vi "GPI_MODE - Type.vi"(8 "error in (no error)":errorcluster, 11 "GPI_MODE":T1) -> (0 "error out":errorcluster, 3 "GPI_MODE_VALUE":i32)   [LabVIEW 2013]
doc: "<b>GPI port state options</b>\nOFF : Input off.\nTRIGGER : Trigger input.\nEXT_EVENT : External signal input."
uses:
  GPI_MODE.ctl
  C:/Projects/Cameras3.x/xiLib/xiLIB_64bit/xiLIB/xiCamLib/API/x64/xiApi.NETX64.dll
  xiLIB_64bit/xiLIB/xiCamLib/API/x64/xiApi.NETX64.dll
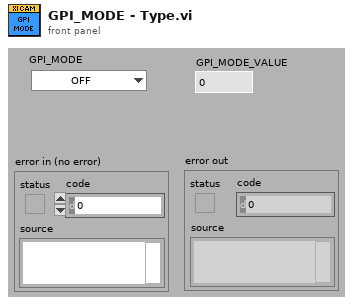
[diagram p1: front panel]
types:
  T1 = typedef "GPI_MODE.ctl" = enum16{"OFF", "TRIGGER", "EXT_EVENT"}
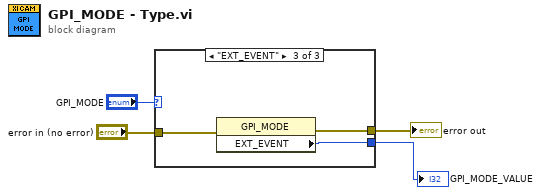
[diagram p0: block diagram]
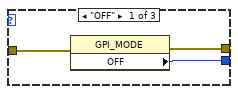
[diagram p2: hidden frame]
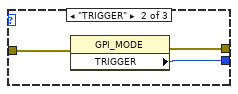
[diagram p3: hidden frame]
diagram:
  n1 = case shown="\"EXT_EVENT\"" "GPI_MODE" {
    tunnel: "error in (no error)" -> [w7 w10 w13]
    tunnel: [w6 w9 w12] -> w2
    tunnel: [w5 w8 w11] -> w1
    frame "OFF" {
      n2 = property class="GPI_MODE"(error in=w7) -> (error out=w6:errorcluster, "OFF"=w5:i32)  [unwired: 1 in, 1 out]
    }
    frame "TRIGGER" {
      n3 = property class="GPI_MODE"(error in=w10) -> (error out=w9:errorcluster, "TRIGGER"=w8:i32)  [unwired: 1 in, 1 out]
    }
    frame "EXT_EVENT" {
      n4 = property class="GPI_MODE"(error in=w13) -> (error out=w12:errorcluster, "EXT_EVENT"=w11:i32)  [unwired: 1 in, 1 out]
    }
  }
  "error out" <- w2
  "GPI_MODE_VALUE" <- w1
